vi "Group History (LV Dbl).vi"(4 "End":dbl, 6 "Start":dbl, 9 "Channels":string[](array[string]), 10 "Group":string, 11 "Historian Module in":refnum<class "Historian Module.lvclass">) -> (2 "Data":T1[](array[typedef]), 3 "Historian Module out":refnum<class "Historian Module.lvclass">)   [LabVIEW 2020, in "VolatusHistorian.lvlib" / "Historian Module.lvclass"]
uses:
  Historian Module.lvclass
  Channel History (LV Dbl).ctl
  Historian Module.lvclass/Historian Module.ctl
  Group Buffer DBL/Group Buffer DBL.lvclass
  VolatusHistorian.lvlib
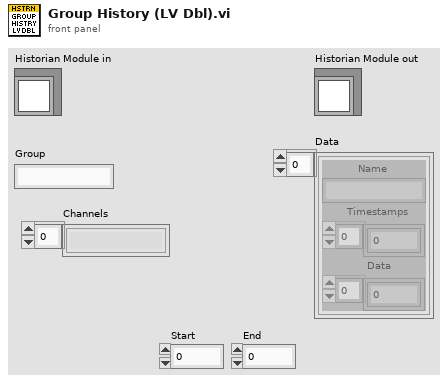
[diagram p1: front panel]
types:
  T1 = typedef "VolatusHistorian.lvlib/Channel History (LV Dbl).ctl" = cluster{"Name":string, "Timestamps":dbl[], "Data":dbl[]}
  T2 = map{string, refnum<class "Group Buffer DBL.lvclass">}
  T3 = typedef "VolatusHistorian.lvlib/Group Data.ctl" = cluster{"Name":string, "Timestamp":dbl[], "Channels":T4[]}
  T4 = typedef "VolatusHistorian.lvlib/Channel Data.ctl" = cluster{"Name":string, "Data":dbl[]}
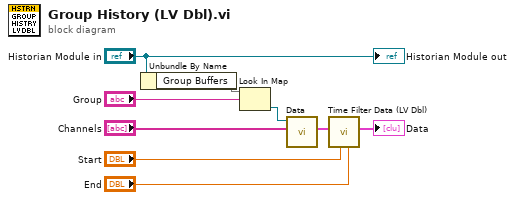
[diagram p0: block diagram]
diagram:
  n1 = Unbundle By Name("Historian Module in") -> ("Group Buffers"=w8:T2)
  n2 = Look In Map(map=w8, key="Group") -> (value=w6:refnum<class "Group Buffer DBL.lvclass">)  [unwired: 1 in, 1 out]
  n3 = call "Data.vi"("Channels (All)"="Channels", "Group Buffer DBL in"=w6) -> ("Group Data"=w4:T3)  [unwired: 7 in, 2 out]
  n4 = call "Time Filter Data (LV Dbl).vi"("End"="End", "Start"="Start", "Group Data"=w4) -> ("Data"=→"Data":T1[])  [unwired: 8 in]
  "Historian Module out" <- "Historian Module in"
